vi "Store Section Text.vi"(6 "Footer":string[](array[string]), 9 "Main Body":string[](array[string]), 10 "End of Header":string[](array[string]), 11 "Section Data in":T2) -> (3 "Section Data out":T2)   [LabVIEW 2018, in "Receipt Parsing.lvlib"]
uses:
  Receipt Parsing.lvlib
  Section Info--cluster.ctl
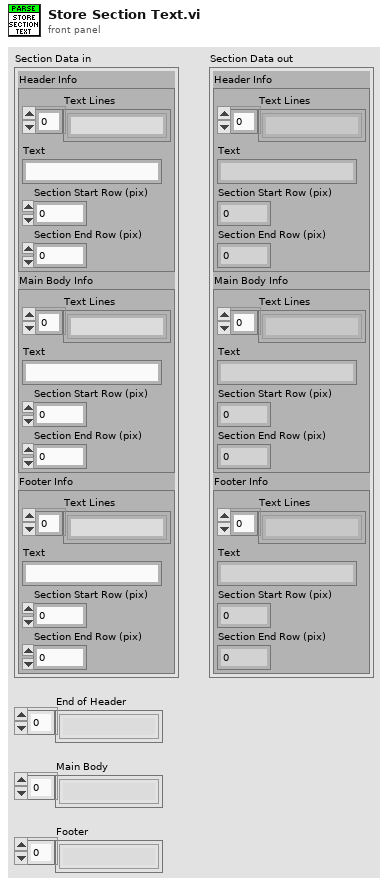
[diagram p1: front panel]
types:
  T1 = typedef "Receipt Parsing.lvlib/Section Info--cluster.ctl" = cluster{"Text Lines":string[], "Text":string, "Section Start Row (pix)":i32, "Section End Row (pix)":i32}
  T2 = cluster{"Header Info":T1, "Main Body Info":T1, "Footer Info":T1}
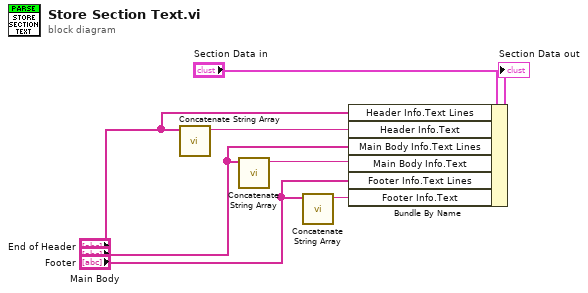
[diagram p0: block diagram]
diagram:
  n1 = call "Concatenate String Array.vi"("Array"="End of Header") -> ("Concatenated String"=w3:string)  [unwired: 10 in]
  n2 = call "Concatenate String Array.vi"("Array"="Main Body") -> ("Concatenated String"=w6:string)  [unwired: 10 in]
  n3 = call "Concatenate String Array.vi"("Array"="Footer") -> ("Concatenated String"=w8:string)  [unwired: 10 in]
  n4 = Bundle By Name(cluster="Section Data in", "Header Info.Text Lines"="End of Header", "Header Info.Text"=w3, "Main Body Info.Text Lines"="Main Body", "Main Body Info.Text"=w6, "Footer Info.Text Lines"="Footer", "Footer Info.Text"=w8) -> (→"Section Data out":T2)
